vi "bundle cluster.vi"(1 "Array 3":dbl[][](array[numeric])) -> (9 "output cluster":T1={"LH"={"Go Up"={"Min Speed"=120.0, "Max Speed"=10.0, "Min Time"=1.82, "Max Time"=3.7, "Min Run Current"=0.0, "Max Run Current"=10.0, "Min Stall Current"=0.0, "Max Stall Current"=25.0, "Min Stall Force"=170.0, "Max Stall Force"=320.0, "Min Stroke"=170.0, "Max Stroke"=320.0}, "Go Down"={"Min Speed"=10.0, "Max Speed"=250.0, "Min Travel Time"=1.82, "Max Travel Time"=3.7, "Min Run Current"=0.0, "Max Run Current"=10.0}, "Shipping"={"Min Distance"=150.0, "Max Distance"=300.0, "Setpoint"=5.0}, "Anti-Pinch"={"Min Force"=5.0, "Max Force"=15.0}}, "RH"={"Go Up"={"Min Speed"=120.0, "Max Speed"=10.0, "Min Time"=1.82, "Max Time"=3.7, "Min Run Current"=0.0, "Max Run Current"=10.0, "Min Stall Current"=0.0, "Max Stall Current"=25.0, "Min Stall Force"=170.0, "Max Stall Force"=320.0, "Min Stroke"=170.0, "Max Stroke"=320.0}, "Go Down"={"Min Speed"=10.0, "Max Speed"=250.0, "Min Travel Time"=1.82, "Max Travel Time"=3.7, "Min Run Current"=0.0, "Max Run Current"=10.0}, "Shipping"={"Min Distance"=150.0, "Max Distance"=300.0, "Setpoint"=5.0}, "Anti-Pinch"={"Min Force"=5.0, "Max Force"=15.0}}, "W 601 FR RH Std"={"Go Up"={"Min Speed"=10.0, "Max Speed"=250.0, "Min Time"=0.5, "Max Time"=4.3, "Min Run Current"=0.0, "Max Run Current"=10.0, "Min Stall Current"=0.0, "Max Stall Current"=25.0, "Min Stall Force"=170.0, "Max Stall Force"=320.0, "Min Stroke"=254.4, "Max Stroke"=270.4}, "Go Down"={"Min Speed"=10.0, "Max Speed"=250.0, "Min Travel Time"=0.5, "Max Travel Time"=4.3, "Min Run Current"=0.0, "Max Run Current"=10.0}, "Shipping"={"Min Distance"=5.0, "Max Distance"=15.0, "Setpoint"=5.0}, "Anti-Pinch"={"Min Force"=5.0, "Max Force"=15.0}}, "W 601 FR LH Std"={"Go Up"={"Min Speed"=10.0, "Max Speed"=250.0, "Min Time"=0.5, "Max Time"=4.3, "Min Run Current"=0.0, "Max Run Current"=10.0, "Min Stall Current"=0.0, "Max Stall Current"=25.0, "Min Stall Force"=170.0, "Max Stall Force"=320.0, "Min Stroke"=254.4, "Max Stroke"=270.4}, "Go Down"={"Min Speed"=10.0, "Max Speed"=250.0, "Min Travel Time"=0.5, "Max Travel Time"=4.3, "Min Run Current"=0.0, "Max Run Current"=10.0}, "Shipping"={"Min Distance"=5.0, "Max Distance"=15.0, "Setpoint"=5.0}, "Anti-Pinch"={"Min Force"=5.0, "Max Force"=15.0}}, "W 601 RR RH Std"={"Go Up"={"Min Speed"=10.0, "Max Speed"=250.0, "Min Time"=0.5, "Max Time"=4.3, "Min Run Current"=0.0, "Max Run Current"=10.0, "Min Stall Current"=0.0, "Max Stall Current"=25.0, "Min Stall Force"=170.0, "Max Stall Force"=320.0, "Min Stroke"=254.4, "Max Stroke"=270.4}, "Go Down"={"Min Speed"=10.0, "Max Speed"=250.0, "Min Travel Time"=0.5, "Max Travel Time"=4.3, "Min Run Current"=0.0, "Max Run Current"=10.0}, "Shipping"={"Min Distance"=5.0, "Max Distance"=15.0, "Setpoint"=5.0}, "Anti-Pinch"={"Min Force"=5.0, "Max Force"=15.0}}, "W 601 RR LH Std"={"Go Up"={"Min Speed"=10.0, "Max Speed"=250.0, "Min Time"=0.5, "Max Time"=4.3, "Min Run Current"=0.0, "Max Run Current"=10.0, "Min Stall Current"=0.0, "Max Stall Current"=25.0, "Min Stall Force"=170.0, "Max Stall Force"=320.0, "Min Stroke"=254.4, "Max Stroke"=270.4}, "Go Down"={"Min Speed"=10.0, "Max Speed"=250.0, "Min Travel Time"=0.5, "Max Travel Time"=4.3, "Min Run Current"=0.0, "Max Run Current"=10.0}, "Shipping"={"Min Distance"=5.0, "Max Distance"=15.0, "Setpoint"=5.0}, "Anti-Pinch"={"Min Force"=5.0, "Max Force"=15.0}}, "W 601 FR RH AP"={"Go Up"={"Min Speed"=10.0, "Max Speed"=250.0, "Min Time"=0.5, "Max Time"=4.3, "Min Run Current"=0.0, "Max Run Current"=10.0, "Min Stall Current"=0.0, "Max Stall Current"=25.0, "Min Stall Force"=170.0, "Max Stall Force"=320.0, "Min Stroke"=254.4, "Max Stroke"=270.4}, "Go Down"={"Min Speed"=10.0, "Max Speed"=250.0, "Min Travel Time"=0.5, "Max Travel Time"=4.3, "Min Run Current"=0.0, "Max Run Current"=10.0}, "Shipping"={"Min Distance"=5.0, "Max Distance"=15.0, "Setpoint"=5.0}, "Anti-Pinch"={"Min Force"=5.0, "Max Force"=15.0}}, "W 601 FR LH AP"={"Go Up"={"Min Speed"=10.0, "Max Speed"=250.0, "Min Time"=0.5, "Max Time"=4.3, "Min Run Current"=0.0, "Max Run Current"=10.0, "Min Stall Current"=0.0, "Max Stall Current"=25.0, "Min Stall Force"=170.0, "Max Stall Force"=320.0, "Min Stroke"=254.4, "Max Stroke"=270.4}, "Go Down"={"Min Speed"=10.0, "Max Speed"=250.0, "Min Travel Time"=0.5, "Max Travel Time"=4.3, "Min Run Current"=0.0, "Max Run Current"=10.0}, "Shipping"={"Min Distance"=5.0, "Max Distance"=15.0, "Setpoint"=5.0}, "Anti-Pinch"={"Min Force"=5.0, "Max Force"=15.0}}, "W 601 RR RH AP"={"Go Up"={"Min Speed"=10.0, "Max Speed"=250.0, "Min Time"=0.5, "Max Time"=4.3, "Min Run Current"=0.0, "Max Run Current"=10.0, "Min Stall Current"=0.0, "Max Stall Current"=25.0, "Min Stall Force"=170.0, "Max Stall Force"=320.0, "Min Stroke"=254.4, "Max Stroke"=270.4}, "Go Down"={"Min Speed"=10.0, "Max Speed"=250.0, "Min Travel Time"=0.5, "Max Travel Time"=4.3, "Min Run Current"=0.0, "Max Run Current"=10.0}, "Shipping"={"Min Distance"=5.0, "Max Distance"=15.0, "Setpoint"=5.0}, "Anti-Pinch"={"Min Force"=5.0, "Max Force"=15.0}}, "W 601 RR LH AP"={"Go Up"={"Min Speed"=10.0, "Max Speed"=250.0, "Min Time"=0.5, "Max Time"=4.3, "Min Run Current"=0.0, "Max Run Current"=10.0, "Min Stall Current"=0.0, "Max Stall Current"=25.0, "Min Stall Force"=170.0, "Max Stall Force"=320.0, "Min Stroke"=254.4, "Max Stroke"=270.4}, "Go Down"={"Min Speed"=10.0, "Max Speed"=250.0, "Min Travel Time"=0.5, "Max Travel Time"=4.3, "Min Run Current"=0.0, "Max Run Current"=10.0}, "Shipping"={"Min Distance"=5.0, "Max Distance"=15.0, "Setpoint"=5.0}, "Anti-Pinch"={"Min Force"=5.0, "Max Force"=15.0}}})   [LabVIEW 2017]
uses:
  controls/All Specs.ctl
  controls/Specifications.ctl
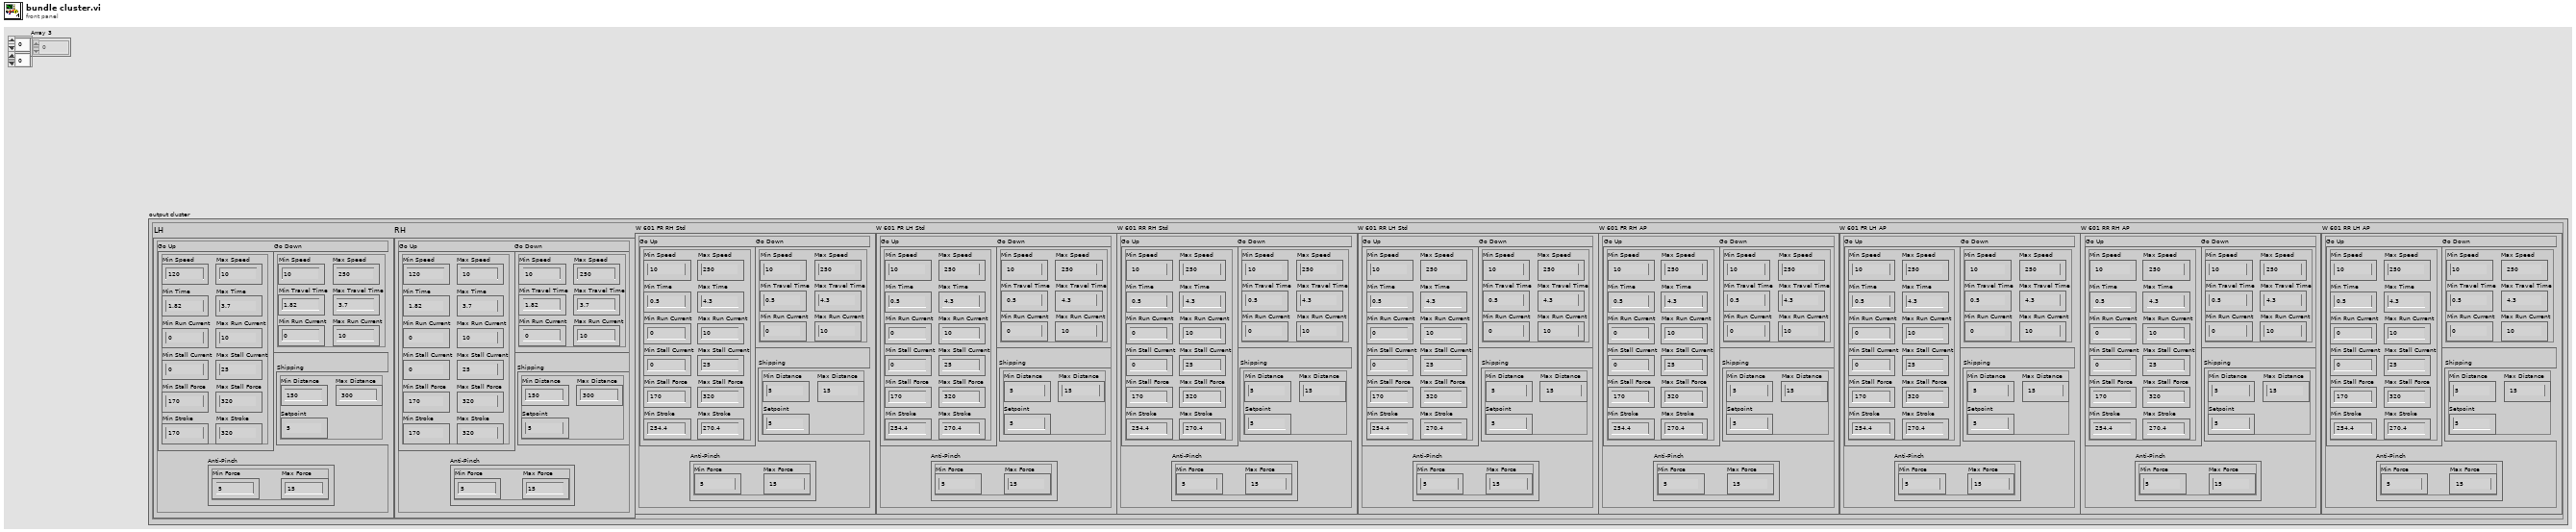
[diagram p1: front panel]
types:
  T1 = typedef "All Specs.ctl" = cluster{"LH":T2, "RH":T2, "W 601 FR RH Std":T2, "W 601 FR LH Std":T2, "W 601 RR RH Std":T2, "W 601 RR LH Std":T2, "W 601 FR RH AP":T2, "W 601 FR LH AP":T2, "W 601 RR RH AP":T2, "W 601 RR LH AP":T2}
  T2 = typedef "Specifications.ctl" = cluster{"Go Up":cluster{"Min Speed":dbl, "Max Speed":dbl, "Min Time":dbl, "Max Time":dbl, "Min Run Current":dbl, "Max Run Current":dbl, "Min Stall Current":dbl, "Max Stall Current":dbl, "Min Stall Force":dbl, "Max Stall Force":dbl, "Min Stroke":dbl, "Max Stroke":dbl}, "Go Down":cluster{"Min Speed":dbl, "Max Speed":dbl, "Min Travel Time":dbl, "Max Travel Time":dbl, "Min Run Current":dbl, "Max Run Current":dbl}, "Shipping":cluster{"Min Distance":dbl, "Max Distance":dbl, "Setpoint":dbl}, "Anti-Pinch":cluster{"Min Force":dbl, "Max Force":dbl}}
  T3 = cluster{"[0]":dbl, "[1]":dbl, "[2]":dbl, "[3]":dbl, "[4]":dbl, "[5]":dbl}
  T4 = cluster{"[0]":dbl, "[1]":dbl, "[2]":dbl, "[3]":dbl, "[4]":dbl, "[5]":dbl, "[6]":dbl, "[7]":dbl, "[8]":dbl, "[9]":dbl, "[10]":dbl, "[11]":dbl}
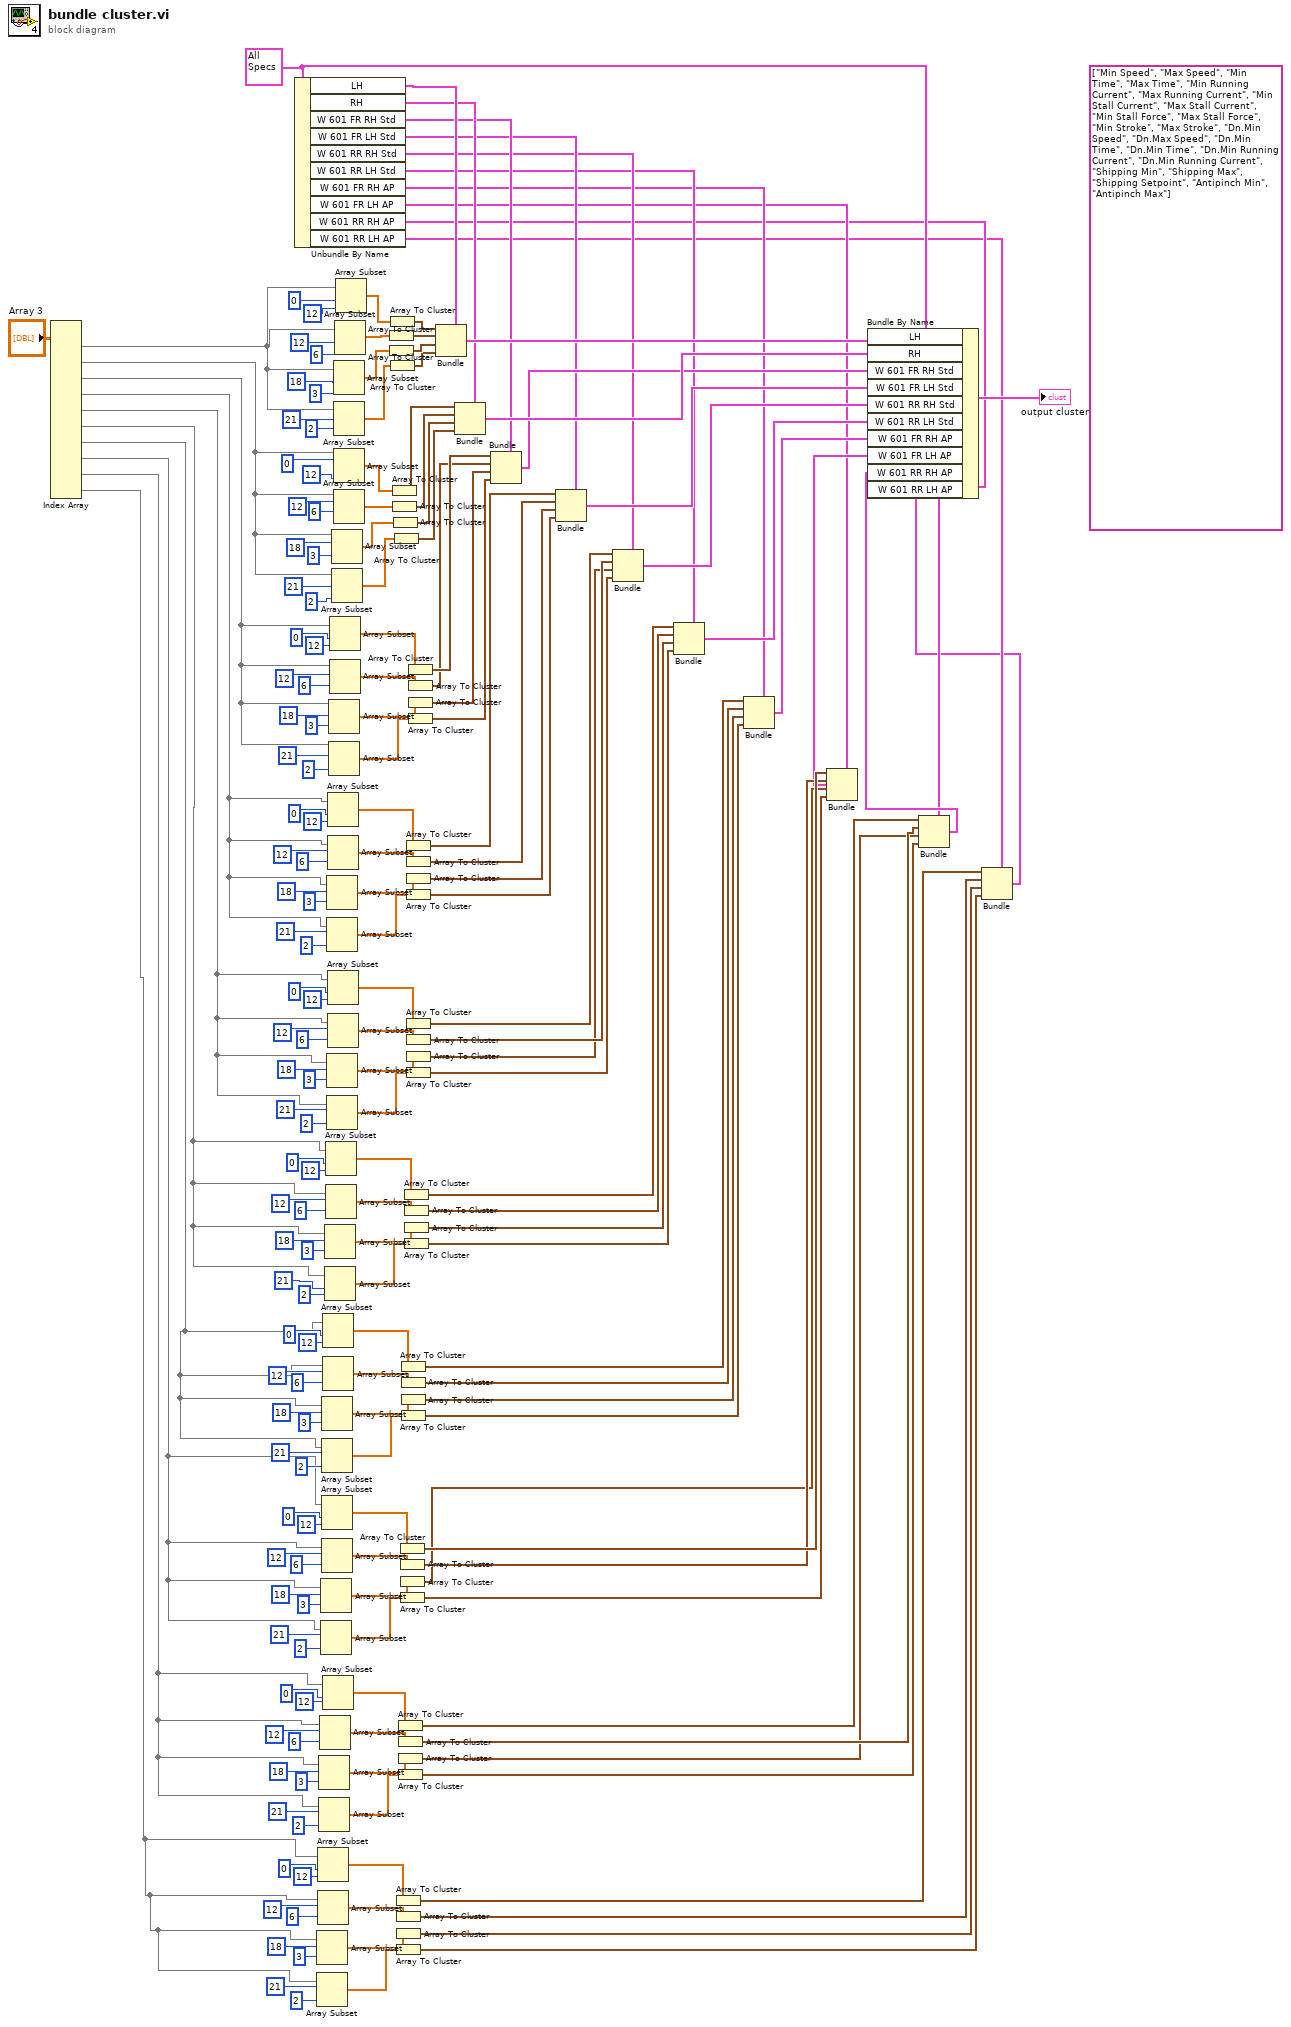
[diagram p0: block diagram]
diagram:
  (unwired) string[] ["Min Speed", "Max Speed", "Min Time", "Max Time", "Min Running Current", "Max Running Current", "Min Stall Current", "Max Stall Current", "Min Stall Force", "Max Stall Force", "Min Stroke", "Max Stroke", "Dn.Min Speed", "Dn.Max Speed", "Dn.Min Time", "Dn.Min Time", "Dn.Min Running Current", "Dn.Min Running Current", "Shipping Min", "Shipping Max", "Shipping Setpoint", "Antipinch Min", "Antipinch Max"]
  w181 = T1 {"LH"={"Go Up"={"Min Speed"=120.0, "Max Speed"=10.0, "Min Time"=1.82, "Max Time"=3.7, "Min Run Current"=0.0, "Max Run Current"=10.0, "Min Stall Current"=0.0, "Max Stall Current"=25.0, "Min Stall Force"=170.0, "Max Stall Force"=320.0, "Min Stroke"=170.0, "Max Stroke"=320.0}, "Go Down"={"Min Speed"=10.0, "Max Speed"=250.0, "Min Travel Time"=1.82, "Max Travel Time"=3.7, "Min Run Current"=0.0, "Max Run Current"=10.0}, "Shipping"={"Min Distance"=150.0, "Max Distance"=300.0, "Setpoint"=5.0}, "Anti-Pinch"={"Min Force"=5.0, "Max Force"=15.0}}, "RH"={"Go Up"={"Min Speed"=120.0, "Max Speed"=10.0, "Min Time"=1.82, "Max Time"=3.7, "Min Run Current"=0.0, "Max Run Current"=10.0, "Min Stall Current"=0.0, "Max Stall Current"=25.0, "Min Stall Force"=170.0, "Max Stall Force"=320.0, "Min Stroke"=170.0, "Max Stroke"=320.0}, "Go Down"={"Min Speed"=10.0, "Max Speed"=250.0, "Min Travel Time"=1.82, "Max Travel Time"=3.7, "Min Run Current"=0.0, "Max Run Current"=10.0}, "Shipping"={"Min Distance"=150.0, "Max Distance"=300.0, "Setpoint"=5.0}, "Anti-Pinch"={"Min Force"=5.0, "Max Force"=15.0}}, "W 601 FR RH Std"={"Go Up"={"Min Speed"=10.0, "Max Speed"=250.0, "Min Time"=0.5, "Max Time"=4.3, "Min Run Current"=0.0, "Max Run Current"=10.0, "Min Stall Current"=0.0, "Max Stall Current"=25.0, "Min Stall Force"=170.0, "Max Stall Force"=320.0, "Min Stroke"=254.4, "Max Stroke"=270.4}, "Go Down"={"Min Speed"=10.0, "Max Speed"=250.0, "Min Travel Time"=0.5, "Max Travel Time"=4.3, "Min Run Current"=0.0, "Max Run Current"=10.0}, "Shipping"={"Min Distance"=5.0, "Max Distance"=15.0, "Setpoint"=5.0}, "Anti-Pinch"={"Min Force"=5.0, "Max Force"=15.0}}, "W 601 FR LH Std"={"Go Up"={"Min Speed"=10.0, "Max Speed"=250.0, "Min Time"=0.5, "Max Time"=4.3, "Min Run Current"=0.0, "Max Run Current"=10.0, "Min Stall Current"=0.0, "Max Stall Current"=25.0, "Min Stall Force"=170.0, "Max Stall Force"=320.0, "Min Stroke"=254.4, "Max Stroke"=270.4}, "Go Down"={"Min Speed"=10.0, "Max Speed"=250.0, "Min Travel Time"=0.5, "Max Travel Time"=4.3, "Min Run Current"=0.0, "Max Run Current"=10.0}, "Shipping"={"Min Distance"=5.0, "Max Distance"=15.0, "Setpoint"=5.0}, "Anti-Pinch"={"Min Force"=5.0, "Max Force"=15.0}}, "W 601 RR RH Std"={"Go Up"={"Min Speed"=10.0, "Max Speed"=250.0, "Min Time"=0.5, "Max Time"=4.3, "Min Run Current"=0.0, "Max Run Current"=10.0, "Min Stall Current"=0.0, "Max Stall Current"=25.0, "Min Stall Force"=170.0, "Max Stall Force"=320.0, "Min Stroke"=254.4, "Max Stroke"=270.4}, "Go Down"={"Min Speed"=10.0, "Max Speed"=250.0, "Min Travel Time"=0.5, "Max Travel Time"=4.3, "Min Run Current"=0.0, "Max Run Current"=10.0}, "Shipping"={"Min Distance"=5.0, "Max Distance"=15.0, "Setpoint"=5.0}, "Anti-Pinch"={"Min Force"=5.0, "Max Force"=15.0}}, "W 601 RR LH Std"={"Go Up"={"Min Speed"=10.0, "Max Speed"=250.0, "Min Time"=0.5, "Max Time"=4.3, "Min Run Current"=0.0, "Max Run Current"=10.0, "Min Stall Current"=0.0, "Max Stall Current"=25.0, "Min Stall Force"=170.0, "Max Stall Force"=320.0, "Min Stroke"=254.4, "Max Stroke"=270.4}, "Go Down"={"Min Speed"=10.0, "Max Speed"=250.0, "Min Travel Time"=0.5, "Max Travel Time"=4.3, "Min Run Current"=0.0, "Max Run Current"=10.0}, "Shipping"={"Min Distance"=5.0, "Max Distance"=15.0, "Setpoint"=5.0}, "Anti-Pinch"={"Min Force"=5.0, "Max Force"=15.0}}, "W 601 FR RH AP"={"Go Up"={"Min Speed"=10.0, "Max Speed"=250.0, "Min Time"=0.5, "Max Time"=4.3, "Min Run Current"=0.0, "Max Run Current"=10.0, "Min Stall Current"=0.0, "Max Stall Current"=25.0, "Min Stall Force"=170.0, "Max Stall Force"=320.0, "Min Stroke"=254.4, "Max Stroke"=270.4}, "Go Down"={"Min Speed"=10.0, "Max Speed"=250.0, "Min Travel Time"=0.5, "Max Travel Time"=4.3, "Min Run Current"=0.0, "Max Run Current"=10.0}, "Shipping"={"Min Distance"=5.0, "Max Distance"=15.0, "Setpoint"=5.0}, "Anti-Pinch"={"Min Force"=5.0, "Max Force"=15.0}}, "W 601 FR LH AP"={"Go Up"={"Min Speed"=10.0, "Max Speed"=250.0, "Min Time"=0.5, "Max Time"=4.3, "Min Run Current"=0.0, "Max Run Current"=10.0, "Min Stall Current"=0.0, "Max Stall Current"=25.0, "Min Stall Force"=170.0, "Max Stall Force"=320.0, "Min Stroke"=254.4, "Max Stroke"=270.4}, "Go Down"={"Min Speed"=10.0, "Max Speed"=250.0, "Min Travel Time"=0.5, "Max Travel Time"=4.3, "Min Run Current"=0.0, "Max Run Current"=10.0}, "Shipping"={"Min Distance"=5.0, "Max Distance"=15.0, "Setpoint"=5.0}, "Anti-Pinch"={"Min Force"=5.0, "Max Force"=15.0}}, "W 601 RR RH AP"={"Go Up"={"Min Speed"=10.0, "Max Speed"=250.0, "Min Time"=0.5, "Max Time"=4.3, "Min Run Current"=0.0, "Max Run Current"=10.0, "Min Stall Current"=0.0, "Max Stall Current"=25.0, "Min Stall Force"=170.0, "Max Stall Force"=320.0, "Min Stroke"=254.4, "Max Stroke"=270.4}, "Go Down"={"Min Speed"=10.0, "Max Speed"=250.0, "Min Travel Time"=0.5, "Max Travel Time"=4.3, "Min Run Current"=0.0, "Max Run Current"=10.0}, "Shipping"={"Min Distance"=5.0, "Max Distance"=15.0, "Setpoint"=5.0}, "Anti-Pinch"={"Min Force"=5.0, "Max Force"=15.0}}, "W 601 RR LH AP"={"Go Up"={"Min Speed"=10.0, "Max Speed"=250.0, "Min Time"=0.5, "Max Time"=4.3, "Min Run Current"=0.0, "Max Run Current"=10.0, "Min Stall Current"=0.0, "Max Stall Current"=25.0, "Min Stall Force"=170.0, "Max Stall Force"=320.0, "Min Stroke"=254.4, "Max Stroke"=270.4}, "Go Down"={"Min Speed"=10.0, "Max Speed"=250.0, "Min Travel Time"=0.5, "Max Travel Time"=4.3, "Min Run Current"=0.0, "Max Run Current"=10.0}, "Shipping"={"Min Distance"=5.0, "Max Distance"=15.0, "Setpoint"=5.0}, "Anti-Pinch"={"Min Force"=5.0, "Max Force"=15.0}}} ("output cluster")
  n1 = Index Array(array="Array 3") -> (element #1=w163:dbl[], element #2=w158:dbl[], element #3=w153:dbl[], element #4=w50:dbl[], element #5=w49:dbl[], element #6=w48:dbl[], element #7=w46:dbl[], element #8=w45:dbl[], element #9=w44:dbl[], element #10=w43:dbl[])  [unwired: 20 in]
  n2 = Unbundle By Name(w181) -> ("LH"=w190:T2, "RH"=w176:T2, "W 601 FR RH Std"=w144:T2, "W 601 FR LH Std"=w8:T2, "W 601 RR RH Std"=w7:T2, "W 601 RR LH Std"=w6:T2, "W 601 FR RH AP"=w5:T2, "W 601 FR LH AP"=w4:T2, "W 601 RR RH AP"=w3:T2, "W 601 RR LH AP"=w2:T2)
  n3 = Array Subset(array=w43, index=18, length=3) -> (w53:dbl[])
  n4 = Array Subset(array=w43, index=21, length=2) -> (w54:dbl[])
  n5 = Array Subset(array=w43, index=0, length=12) -> (w51:dbl[])
  n6 = Array Subset(array=w43, index=12, length=6) -> (w52:dbl[])
  n7 = Array Subset(array=w44, index=18, length=3) -> (w72:dbl[])
  n8 = Array Subset(array=w44, index=21, length=2) -> (w71:dbl[])
  n9 = Array Subset(array=w44, index=12, length=6) -> (w73:dbl[])
  n10 = Array Subset(array=w45, index=18, length=3) -> (w77:dbl[])
  n11 = Array Subset(array=w45, index=21, length=2) -> (w78:dbl[])
  n12 = Array Subset(array=w46, index=18, length=3) -> (w96:dbl[])
  n13 = Array Subset(array=w46, index=21, length=2) -> (w95:dbl[])
  n14 = Array Subset(array=w45, index=0, length=12) -> (w75:dbl[])
  n15 = Array Subset(array=w45, index=12, length=6) -> (w76:dbl[])
  n16 = Array Subset(array=w46, index=0, length=12) -> (w98:dbl[])
  n17 = Array Subset(array=w46, index=12, length=6) -> (w97:dbl[])
  n18 = Array Subset(array=w44, index=0, length=12) -> (w74:dbl[])
  n19 = Array Subset(array=w48, index=18, length=3) -> (w101:dbl[])
  n20 = Array Subset(array=w48, index=21, length=2) -> (w102:dbl[])
  n21 = Array Subset(array=w48, index=0, length=12) -> (w99:dbl[])
  n22 = Array Subset(array=w48, index=12, length=6) -> (w100:dbl[])
  n23 = Array Subset(array=w50, index=18, length=3) -> (w124:dbl[])
  n24 = Array Subset(array=w50, index=21, length=2) -> (w125:dbl[])
  n25 = Array Subset(array=w49, index=18, length=3) -> (w119:dbl[])
  n26 = Array Subset(array=w49, index=21, length=2) -> (w118:dbl[])
  n27 = Array Subset(array=w50, index=0, length=12) -> (w122:dbl[])
  n28 = Array Subset(array=w50, index=12, length=6) -> (w123:dbl[])
  n29 = Array Subset(array=w49, index=0, length=12) -> (w121:dbl[])
  n30 = Array Subset(array=w49, index=12, length=6) -> (w120:dbl[])
  n31 = Array Subset(array=w153, index=18, length=3) -> (w150:dbl[])
  n32 = Array Subset(array=w153, index=21, length=2) -> (w149:dbl[])
  n33 = Array Subset(array=w153, index=0, length=12) -> (w152:dbl[])
  n34 = Array Subset(array=w153, index=12, length=6) -> (w151:dbl[])
  n35 = Array Subset(array=w158, index=18, length=3) -> (w175:dbl[])
  n36 = Array Subset(array=w158, index=21, length=2) -> (w155:dbl[])
  n37 = Array Subset(array=w163, index=18, length=3) -> (w184:dbl[])
  n38 = Array Subset(array=w163, index=21, length=2) -> (w160:dbl[])
  n39 = Array Subset(array=w158, index=0, length=12) -> (w170:dbl[])
  n40 = Array Subset(array=w158, index=12, length=6) -> (w173:dbl[])
  n41 = Array Subset(array=w163, index=12, length=6) -> (w187:dbl[])
  n42 = Array Subset(array=w163, index=0, length=12) -> (w191:dbl[])
  n43 = Array To Cluster(array=w187) -> (cluster=w179:T3)
  n44 = Array To Cluster(array=w184) -> (cluster=w178:cluster{"[0]":dbl, "[1]":dbl, "[2]":dbl})
  n45 = Array To Cluster(array=w191) -> (cluster=w180:T4)
  n46 = Array To Cluster(array=w160) -> (cluster=w159:cluster{"[0]":dbl, "[1]":dbl})
  n47 = Array To Cluster(array=w170) -> (cluster=w167:T4)
  n48 = Array To Cluster(array=w173) -> (cluster=w166:T3)
  n49 = Array To Cluster(array=w175) -> (cluster=w165:cluster{"[0]":dbl, "[1]":dbl, "[2]":dbl})
  n50 = Array To Cluster(array=w155) -> (cluster=w154:cluster{"[0]":dbl, "[1]":dbl})
  n51 = Array To Cluster(array=w51) -> (cluster=w18:T4)
  n52 = Array To Cluster(array=w52) -> (cluster=w17:T3)
  n53 = Array To Cluster(array=w53) -> (cluster=w16:cluster{"[0]":dbl, "[1]":dbl, "[2]":dbl})
  n54 = Array To Cluster(array=w54) -> (cluster=w15:cluster{"[0]":dbl, "[1]":dbl})
  n55 = Array To Cluster(array=w74) -> (cluster=w22:T4)
  n56 = Array To Cluster(array=w73) -> (cluster=w21:T3)
  n57 = Array To Cluster(array=w72) -> (cluster=w20:cluster{"[0]":dbl, "[1]":dbl, "[2]":dbl})
  n58 = Array To Cluster(array=w71) -> (cluster=w19:cluster{"[0]":dbl, "[1]":dbl})
  n59 = Array To Cluster(array=w75) -> (cluster=w26:T4)
  n60 = Array To Cluster(array=w76) -> (cluster=w25:T3)
  n61 = Array To Cluster(array=w77) -> (cluster=w24:cluster{"[0]":dbl, "[1]":dbl, "[2]":dbl})
  n62 = Array To Cluster(array=w78) -> (cluster=w23:cluster{"[0]":dbl, "[1]":dbl})
  n63 = Array To Cluster(array=w98) -> (cluster=w30:T4)
  n64 = Array To Cluster(array=w97) -> (cluster=w29:T3)
  n65 = Array To Cluster(array=w96) -> (cluster=w28:cluster{"[0]":dbl, "[1]":dbl, "[2]":dbl})
  n66 = Array To Cluster(array=w95) -> (cluster=w27:cluster{"[0]":dbl, "[1]":dbl})
  n67 = Array To Cluster(array=w99) -> (cluster=w34:T4)
  n68 = Array To Cluster(array=w100) -> (cluster=w33:T3)
  n69 = Array To Cluster(array=w101) -> (cluster=w32:cluster{"[0]":dbl, "[1]":dbl, "[2]":dbl})
  n70 = Array To Cluster(array=w102) -> (cluster=w31:cluster{"[0]":dbl, "[1]":dbl})
  n71 = Array To Cluster(array=w122) -> (cluster=w42:T4)
  n72 = Array To Cluster(array=w123) -> (cluster=w41:T3)
  n73 = Array To Cluster(array=w124) -> (cluster=w40:cluster{"[0]":dbl, "[1]":dbl, "[2]":dbl})
  n74 = Array To Cluster(array=w125) -> (cluster=w39:cluster{"[0]":dbl, "[1]":dbl})
  n75 = Array To Cluster(array=w121) -> (cluster=w38:T4)
  n76 = Array To Cluster(array=w120) -> (cluster=w37:T3)
  n77 = Array To Cluster(array=w119) -> (cluster=w36:cluster{"[0]":dbl, "[1]":dbl, "[2]":dbl})
  n78 = Array To Cluster(array=w118) -> (cluster=w35:cluster{"[0]":dbl, "[1]":dbl})
  n79 = Array To Cluster(array=w152) -> (cluster=w148:T4)
  n80 = Array To Cluster(array=w151) -> (cluster=w147:T3)
  n81 = Array To Cluster(array=w150) -> (cluster=w146:cluster{"[0]":dbl, "[1]":dbl, "[2]":dbl})
  n82 = Array To Cluster(array=w149) -> (cluster=w145:cluster{"[0]":dbl, "[1]":dbl})
  n83 = Bundle(cluster=w190, "Go Up"=w180, "Go Down"=w179, "Shipping"=w178, "Anti-Pinch"=w159) -> (w183:T2)
  n84 = Bundle(cluster=w176, "Go Up"=w167, "Go Down"=w166, "Shipping"=w165, "Anti-Pinch"=w154) -> (w182:T2)
  n85 = Bundle(cluster=w144, "Go Up"=w148, "Go Down"=w147, "Shipping"=w146, "Anti-Pinch"=w145) -> (w143:T2)
  n86 = Bundle(cluster=w8, "Go Up"=w42, "Go Down"=w41, "Shipping"=w40, "Anti-Pinch"=w39) -> (w14:T2)
  n87 = Bundle(cluster=w7, "Go Up"=w38, "Go Down"=w37, "Shipping"=w36, "Anti-Pinch"=w35) -> (w13:T2)
  n88 = Bundle(cluster=w6, "Go Up"=w34, "Go Down"=w33, "Shipping"=w32, "Anti-Pinch"=w31) -> (w12:T2)
  n89 = Bundle(cluster=w5, "Go Up"=w30, "Go Down"=w29, "Shipping"=w28, "Anti-Pinch"=w27) -> (w11:T2)
  n90 = Bundle(cluster=w4, "Go Up"=w26, "Go Down"=w25, "Shipping"=w24, "Anti-Pinch"=w23) -> (w10:T2)
  n91 = Bundle(cluster=w3, "Go Up"=w22, "Go Down"=w21, "Shipping"=w20, "Anti-Pinch"=w19) -> (w9:T2)
  n92 = Bundle(cluster=w2, "Go Up"=w18, "Go Down"=w17, "Shipping"=w16, "Anti-Pinch"=w15) -> (w1:T2)
  n93 = Bundle By Name(cluster=w181, "LH"=w183, "RH"=w182, "W 601 FR RH Std"=w143, "W 601 FR LH Std"=w14, "W 601 RR RH Std"=w13, "W 601 RR LH Std"=w12, "W 601 FR RH AP"=w11, "W 601 FR LH AP"=w10, "W 601 RR RH AP"=w9, "W 601 RR LH AP"=w1) -> (→"output cluster":T1)
